vi "SweepSetup.vi"(0 "VISA IN":refnum<visa-resource-name>, 1 "Source Frq. Mode":string(combo)="STEPped", 2 "Dwell Time(sec)":dbl, 3 "Alternate Sweeps?":bool, 5 "error in":errorcluster, 7 "Channel":i32=1) -> (14 "VISA Out":refnum<visa-resource-name>, 19 "error out":errorcluster)   [LabVIEW 2018, in "PNA-X.lvlib"]
uses:
  PNA-X.lvlib
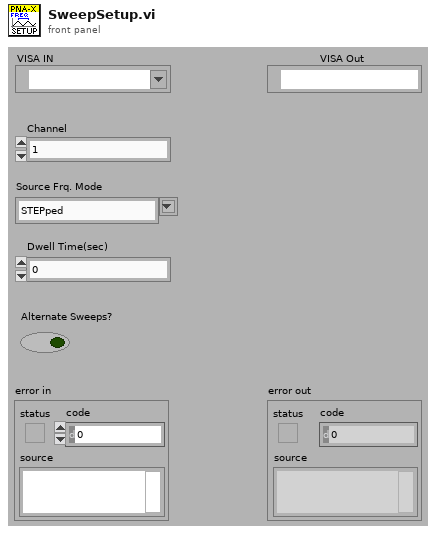
[diagram p1: front panel]
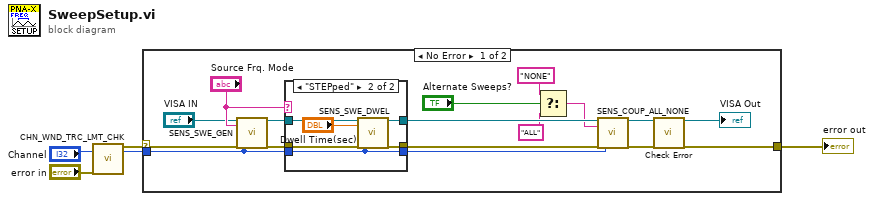
[diagram p0: block diagram]
diagram:
  n1 = call "CHN_WND_TRC_LMT_CHK.vi"("Channel"="Channel", "error in"="error in") -> ("error out"=w4:errorcluster, "Channel"=w3:i32)  [unwired: 13 in, 3 out]
  n2 = case shown="No Error" w4 {
    selector: w4 -> [w19 w32]
    tunnel: w3 -> [w18 _]
    tunnel: [w15 w32] -> w2
    frame No Error {
      n3 = call "SENS_SWE_GEN.vi"("VISA IN"="VISA IN", "Source Frq. Mode"="Source Frq. Mode", "error in"=w19, "Channel"=w18) -> ("VISA Out"=w21:refnum<visa-resource-name>, "error out"=w20:errorcluster)  [unwired: 14 in]
      n4 = case shown="\"STEPped\"" "Source Frq. Mode" {
        tunnel: w20 -> [w24 w31]
        tunnel: [w24 w30] -> w13
        tunnel: w21 -> [w25 w29]
        tunnel: [w25 w28] -> w14
        tunnel: w18 -> [w23 w26]
        tunnel: [w23 w26] -> w10
        frame Default {
        }
        frame "STEPped" {
          n5 = call "SENS_SWE_DWEL.vi"("VISA IN"=w29, "Dwell Time(sec)"="Dwell Time(sec)", "error in"=w31, "Channel"=w26) -> ("VISA Out"=w28:refnum<visa-resource-name>, "error out"=w30:errorcluster)  [unwired: 14 in]
        }
      }
      n6 = Select(t="NONE" ("Sweep Mode(ALL or NONE)"), s="Alternate Sweeps?", f="ALL" ("Sweep Mode(ALL or NONE)")) -> (s? t:f=w6:string)
      n7 = call "SENS_COUP_ALL_NONE.vi"("VISA IN"=w14, "Sweep Mode(ALL or NONE)"=w6, "error in"=w13, "Channel"=w10) -> ("VISA Out"=w12:refnum<visa-resource-name>, "error out"=w11:errorcluster)  [unwired: 14 in]
      n8 = call "Check Error.vi"("VISA Resource Name"=w12, "error in (no error)"=w11) -> ("dup VISA session"=→"VISA Out":refnum<visa-resource-name>, "error out"=w15:errorcluster)  [unwired: 16 in]
    }
    frame Error {
    }
  }
  "error out" <- w2
